vi "Auto Fill.vi"(6 "Use .txt file":bool=TRUE, 7 "group name":string="Untitled", 8 "Error In":errorcluster, 9 "X column name":string="Field_fixed", 10 "Channel info":T1[](array[typedef]) caption="Channel                   pts per sine    phase", 11 "Data file path":path=path "C:/Data/October_2012/100112/s004_100112.tdms") -> (0 "Error Out":errorcluster, 1 "X column name out":string="Field_fixed", 2 "Channel info out":T1[](array[typedef]) caption="Channel                   pts per sine    phase", 3 "Data file path out":path=path "C:/Data/October_2012/100112/s004_100112.tdms")   [LabVIEW 2015]
uses:
  CH_name_pts_phase.ctl
panel:
  out "File channel names":string[](array[string])
  out "points":i32[](array[numeric])
  out "Channels":string[](array[string])
  out "text":string
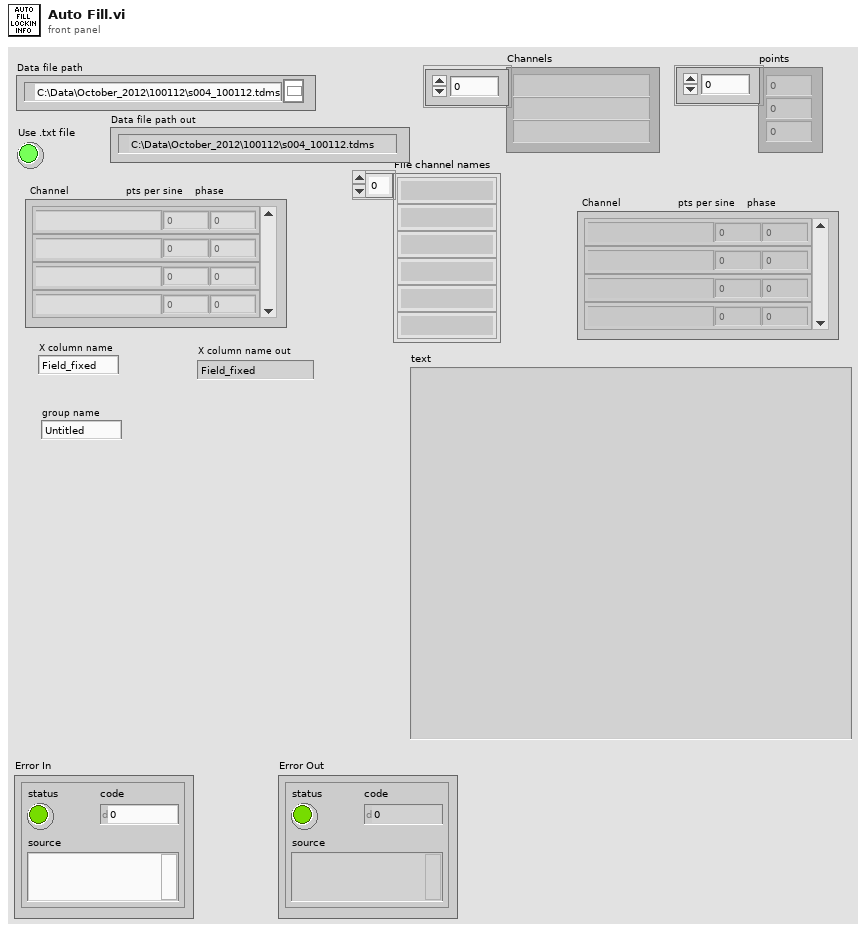
[diagram p1: front panel]
types:
  T1 = typedef "CH_name_pts_phase.ctl" = cluster{"Channel":string, "pts per sine wave":i32, "Phase":dbl}
  T2 = enum16{"open", "open or create", "create or replace", "create", "open (read-only)"}
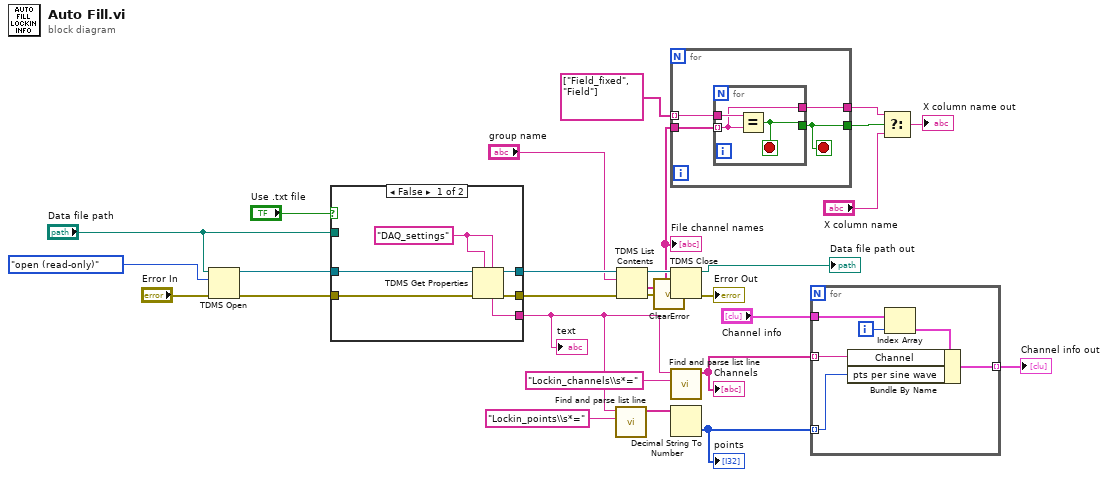
[diagram p0: block diagram]
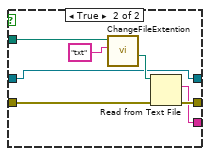
[diagram p2: hidden frame]
diagram:
  n1 = TDMS Open(8:"Error In", 10:T2."open (read-only)" ("operation (0:open)"), 11:"Data file path") -> (0:w25:errorcluster, 3:w27:refnum<k34>)  [unwired: 4 in]
  n2 = case shown="False" "Use .txt file" {
    tunnel: w27 -> [w34 w36]
    tunnel: [w33 w36] -> w26
    tunnel: [w32 w37] -> w11
    tunnel: w25 -> [w31 w39]
    tunnel: "Data file path" -> [_ w38]
    tunnel: [w29 w35] -> w21
    frame False {
      w30 = "DAQ_settings" ("property name")
      n3 = TDMS Get Properties(5:w30, 7:w30, 8:w31, 11:w34) -> (0:w32:errorcluster, 3:w33:refnum<k34>, 4:w29:string)  [unwired: 2 in, 3 out]
    }
    frame True {
      n4 = call "ChangeFileExtention.vi"("New Extention"="txt", "Path"=w38) -> ("Path with new extension"=w41:path)  [unwired: 1 in, 8 out]
      n5 = Read from Text File(file (use dialog)=w41, error in=w39) -> (text=w35:string, error out=w37:errorcluster)  [unwired: 2 in, 2 out]
    }
  }
  "text" <- w21
  n6 = call "Find and parse list line.vi"("Property"="Lockin_points\\s*=" ("regular expression"), "String"=w21) -> ("List"=w19:string[])  [unwired: 8 in, 1 out]
  n7 = TDMS List Contents(4:w11, 6:"group name", 7:w26) -> (0:w1:errorcluster, 1:w8:string[], 3:w12:refnum<k34>)  [unwired: 1 out]
  "File channel names" <- w8
  n8 = call <vilib>:"ClearError.vi"("error in (no error)"=w1) -> ("error out"=w10:errorcluster)
  n9 = for {
    tunnel: w8 -> [w45]
    tunnel: string[] ["Field_fixed", "Field"] ("channel names") -> [w44] mode=indexing
    tunnel: [w42] -> w5
    tunnel: [w43] -> w6
    stop <- w43 stop-if-true
    n10 = for {
      tunnel: w45 -> [w46] mode=indexing
      tunnel: w44 -> [w48]
      tunnel: [w47] -> w43
      tunnel: [w46] -> w42
      stop <- w47 stop-if-true
      n11 = Equal?(x=w48, y=w46) -> (x = y?=w47:bool)
    }
  }
  n12 = TDMS Close(8:w10, 11:w12) -> (0:→"Error Out":errorcluster, 3:→"Data file path out":path)
  n13 = call "Find and parse list line.vi"("Property"="Lockin_channels\\s*=" ("regular expression"), "String"=w21) -> ("List"=w17:string[])  [unwired: 8 in, 1 out]
  "Channels" <- w17
  n14 = Decimal String To Number(string=w19) -> (number=w16:i32[])  [unwired: 2 in, 1 out]
  "points" <- w16
  n15 = for {
    tunnel: "Channel info" -> [w54]
    tunnel: w17 -> [w52] mode=indexing
    tunnel: w16 -> [w51] mode=indexing
    tunnel: [w49] -> w15 mode=indexing
    i -> [w53]
    n16 = Index Array(array=w54, index=w53) -> (element=w50:T1)
    n17 = Bundle By Name(cluster=w50, "Channel"=w52, "pts per sine wave"=w51) -> (w49:T1)
  }
  "Channel info out" <- w15
  n18 = Select(t=w5, s=w6, f="X column name") -> (s? t:f=→"X column name out":string)
